vi "Set Screw.vi"(8 "error in (no error)":errorcluster, 9 "Enabled?":T1(ring), 10 "Screw":u16(ring)=1 items=["0%"=1, "25%"=225, "50%"=450, "75%"=675, "100%"=900], 11 "Feeder Actor.lvlib:Screw.lvclass":refnum<class "Screw.lvclass">) -> (0 "error out":errorcluster, 3 "Actor out":refnum<class "Actor.lvclass">)   [LabVIEW 2018, in "Feeder Actor.lvlib" / "Screw.lvclass"]
uses:
  Screw.lvclass
  <vilib>/ActorFramework/Actor/Actor.lvclass
  C:/Program Files/National Instruments/LabVIEW 2018/vi.lib/ActorFramework/Actor/Actor.lvclass
  Screw.lvclass/Screw.ctl
  <resource>/objmgr/daqmx.rc
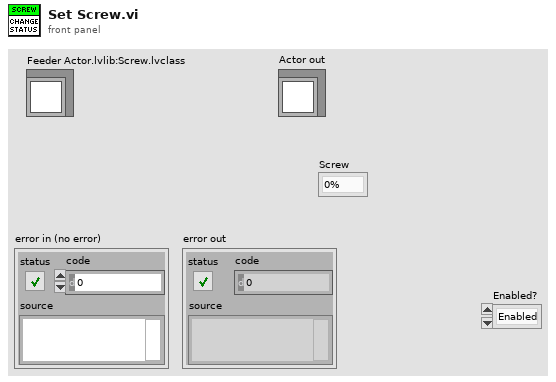
[diagram p1: front panel]
types:
  T1 = enum8{"Enabled", "Disabled", "Disabled and Grayed Out"}
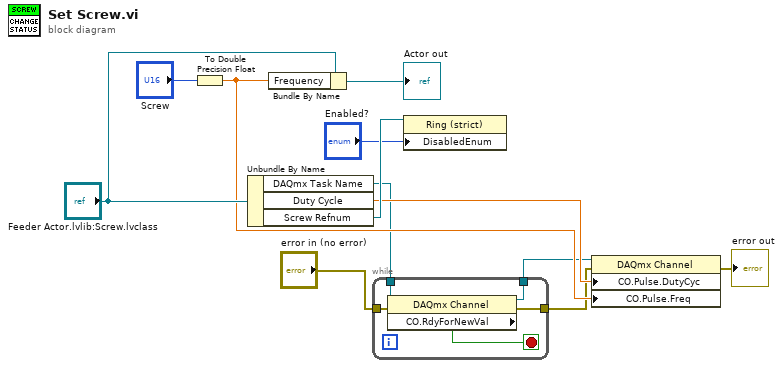
[diagram p0: block diagram]
diagram:
  n1 = To Double Precision Float(number="Screw") -> (double precision float=w6:dbl)
  n2 = Unbundle By Name("Feeder Actor.lvlib:Screw.lvclass") -> ("DAQmx Task Name"=w3:refnum<k21>, "Duty Cycle"=w7:dbl, "Screw Refnum"=w10:refnum<vi>)
  n3 = Bundle By Name(cluster="Feeder Actor.lvlib:Screw.lvclass", "Frequency"=w6) -> (→"Actor out":refnum<class "Screw.lvclass">)
  n4 = while {
    tunnel: "error in (no error)" -> [w17]
    tunnel: w3 -> [w16]
    tunnel: [w14] -> w2
    tunnel: [w13] -> w1
    stop <- w15 stop-if-true
    n5 = property class="DAQmx Channel"(reference=w16, error in=w17) -> (reference out=w14:refnum<k21>, error out=w13:errorcluster, "CO.RdyForNewVal"=w15:bool)
  }
  n6 = property class="Ring (strict)"(reference=w10, "DisabledEnum"="Enabled?") -> ()  [unwired: 1 in, 2 out]
  n7 = property class="DAQmx Channel"(reference=w2, error in=w1, "CO.Pulse.DutyCyc"=w7, "CO.Pulse.Freq"=w6) -> (error out=→"error out":errorcluster)  [unwired: 1 out]
